vi "DAQmx Create Channel (AI-Voltage-Basic).vi"(0 "task in":refnum<k21>, 1 "maximum value":dbl=5.0 format="%0.2f", 2 "minimum value":dbl=-5.0 format="%0.2f", 3 "input terminal configuration":i32(ring)=-1 items=["default"=-1, "RSE"=10083, "NRSE"=10078, "Differential"=10106, "Pseudodifferential"=12529], 5 "physical channels":tag, 7 "name to assign":string, 9 "units":i32(ring)=10348 items=["Volts"=10348, "From Custom Scale"=10065], 11 "error in":errorcluster, 12 "custom scale name":tag) -> (4 "task out":refnum<k21>, 15 "error out":errorcluster)   [LabVIEW 2013]
doc: "Creates channel(s) to measure voltage. If the measurement requires the use of internal excitation or you need excitation to scale the voltage, use the AI Custom Voltage with Excitation instance of this VI."
uses:
  C:/Program Files/National Instruments/LabVIEW 2013/resource/objmgr/daqmx.rc
panel:
  # "input limits"
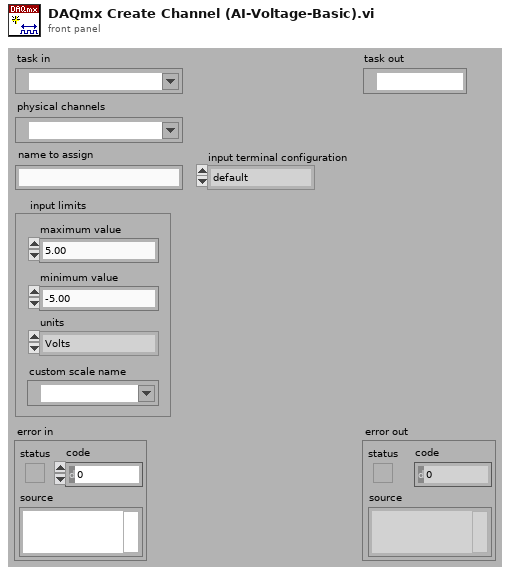
[diagram p1: front panel]
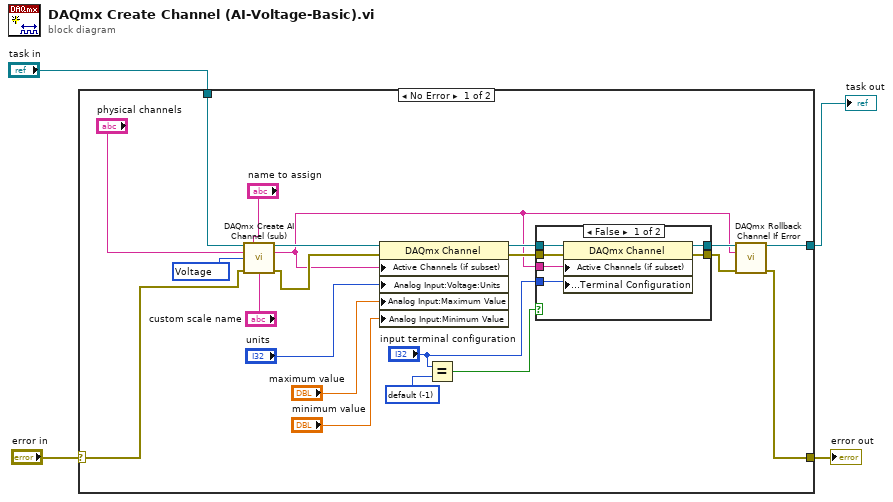
[diagram p0: block diagram]
diagram:
  n1 = case shown="No Error" "error in" {
    selector: "error in" -> [w24 w35]
    tunnel: [w6 w35] -> w2
    tunnel: "task in" -> [w25 w34]
    tunnel: [w7 w34] -> w1
    frame No Error {
      w13 = -1 items=["default"=-1, "differential"=10106, "RSE"=10083, "NRSE"=10078] ("input terminal configuration")
      w15 = 10322 items=["Voltage"=10322, "Current"=10134, "More:Voltage:Custom with Excitation"=10323, "More:Current:Custom with Excitation"=10136, "Frequency"=10181, "Period"=10257, "Resistance"=10278, "Temperature:Thermocouple"=10303, "Temperature:Thermistor"=10302, "Temperature:RTD"=10301, "Temperature:Built-in Sensor"=10311, "Strain Gage"=10300] ("measurement type")
      n2 = call "DAQmx Create AI Channel (sub).vi"("task in"=w25, "virtual channel name"="name to assign", "physical channel name"="physical channels", "measurement type"=w15, "error in"=w24, "custom scale"="custom scale name") -> ("task out"=w10:refnum<k21>, "channel names"=w5:string, "error out"=w21:errorcluster)  [unwired: 1 in, 6 out]
      n3 = property class="DAQmx Channel"(reference=w10, error in=w21, "Active Channels (if subset)"=w5, "Analog Input:Voltage:Units"="units", "Analog Input:Maximum Value"="maximum value", "Analog Input:Minimum Value"="minimum value") -> (reference out=w11:refnum<k21>, error out=w17:errorcluster)
      n4 = Equal?(x="input terminal configuration", y=w13) -> (x = y?=w18:bool)
      n5 = case shown="False" w18 {
        tunnel: w17 -> [w31 w33]
        tunnel: [w30 w32] -> w9
        tunnel: [w29 w33] -> w8
        tunnel: "input terminal configuration" -> [w28 _]
        tunnel: w5 -> [w27 _]
        tunnel: w11 -> [w26 w32]
        frame False {
          n6 = property class="DAQmx Channel"(reference=w26, error in=w31, "Active Channels (if subset)"=w27, "Analog Input:General Properties:Input Configuration:Terminal Configuration"=w28) -> (reference out=w30:refnum<k21>, error out=w29:errorcluster)
        }
        frame True {
        }
      }
      n7 = call "DAQmx Rollback Channel If Error.vi"("task in"=w9, "channel names"=w5, "error in"=w8) -> ("task out"=w7:refnum<k21>, "error out"=w6:errorcluster)  [unwired: 11 out]
    }
    frame Error {
    }
  }
  "error out" <- w2
  "task out" <- w1
